vi "FT10_Log Create TDMS File.vi"() -> (0 "t0":T1, 2 "tdms file out":T2)   [LabVIEW 2015]
uses:
  Controls/Control_Log TDMS Filename.ctl
  Controls/Control_Log t0.ctl
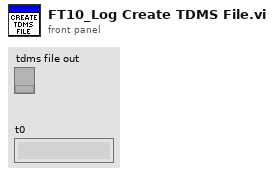
[diagram p1: front panel]
types:
  T1 = typedef "Control_Log t0.ctl" = string
  T2 = typedef "Control_Log TDMS Filename.ctl" = refnum<k34>
  T3 = enum16{"open", "open or create", "create or replace", "create", "open (read-only)"}
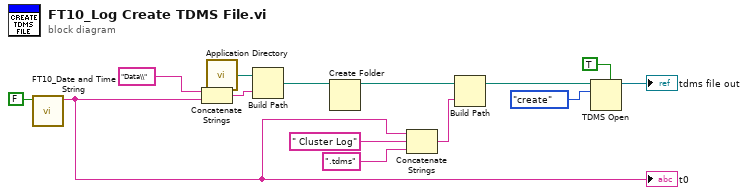
[diagram p0: block diagram]
diagram:
  n1 = call "FT10_Date and Time String.vi"("to UTC"=FALSE) -> ("Date & Time string"=w2:string)  [unwired: 10 in]
  "t0" <- w2
  n2 = Concatenate Strings("Data\\" ("string"), w2) -> (w13:string)
  n3 = call <vilib>:"Application Directory.vi"() -> ("Application Directory"=w12:path)
  n4 = Build Path(base path=w12, name or relative path=w13) -> (appended path=w7:path)
  n5 = Create Folder(path (use dialog)=w7) -> (created path=w6:path)  [unwired: 2 in, 2 out]
  n6 = Concatenate Strings(w2, " Cluster Log" ("name or relative path"), ".tdms" ("string")) -> (w1:string)
  n7 = Build Path(base path=w6, name or relative path=w1) -> (appended path=w3:path)
  n8 = TDMS Open(5:TRUE ("create index file? (T)"), 10:T3."create" ("operation (0:open)"), 11:w3) -> (3:→"tdms file out":refnum<k34>)  [unwired: 4 in, 1 out]
